vi "VI_Info_da_Quadra_Dasboard.vi"() -> (10 "Match_Time":dbl, 12 "Robot_Position":bool, 14 "Scale_L":bool, 15 "Scale_R":bool, 16 "Switch_R":bool, 17 "Switch_L":bool, 19 "Same_Side":bool)   [LabVIEW 2017]
uses:
  <vilib>/Rock Robotics/Network Tables/NT Read String.vi
  <vilib>/Rock Robotics/Network Tables/NT Read Number.vi
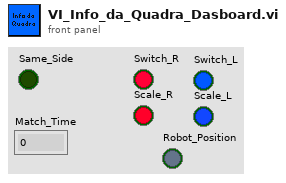
[diagram p1: front panel]
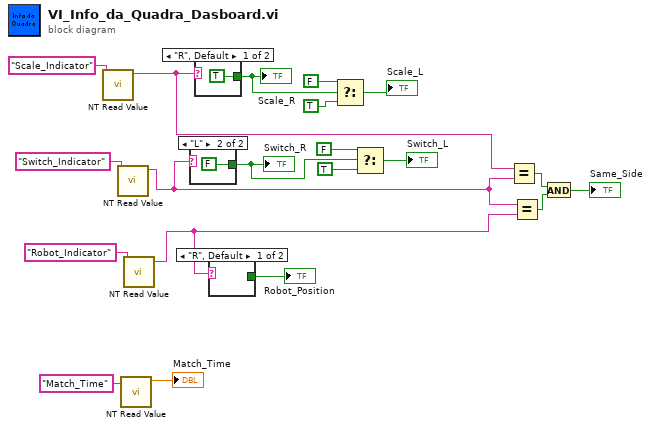
[diagram p0: block diagram]
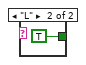
[diagram p2: hidden frame]
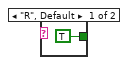
[diagram p3: hidden frame]
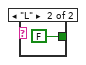
[diagram p4: hidden frame]
diagram:
  n1 = call-poly <vilib>:"NT Read Value.vi"("Name"="Scale_Indicator") -> ("String"=w14:string)  [unwired: 9 in, 1 out]
  n2 = call-poly <vilib>:"NT Read Value.vi"("Name"="Switch_Indicator") -> ("String"=w13:string)  [unwired: 9 in, 1 out]
  n3 = call-poly <vilib>:"NT Read Value.vi"("Name"="Match_Time") -> ("Numeric"=→"Match_Time":dbl)  [unwired: 9 in, 1 out]
  n4 = call-poly <vilib>:"NT Read Value.vi"("Name"="Robot_Indicator") -> ("String"=w12:string)  [unwired: 9 in, 1 out]
  n5 = case shown="\"L\"" w13 {
    tunnel: [TRUE FALSE] -> w8
    frame "R", Default {
    }
    frame "L" {
    }
  }
  "Switch_R" <- w8
  n6 = case shown="\"R\", Default" w14 {
    tunnel: [TRUE FALSE] -> w11
    frame "R", Default {
    }
    frame "L" {
    }
  }
  "Scale_R" <- w11
  n7 = case shown="\"R\", Default" w12 {
    tunnel: [_ TRUE] -> w3
    frame "R", Default {
    }
    frame "L" {
    }
  }
  "Robot_Position" <- w3
  n8 = Select(t=FALSE, s=w11, f=TRUE) -> (s? t:f=→"Scale_L":bool)
  n9 = Select(t=FALSE, s=w8, f=TRUE) -> (s? t:f=→"Switch_L":bool)
  n10 = Equal?(x=w14, y=w13) -> (x = y?=w16:bool)
  n11 = Equal?(x=w13, y=w12) -> (x = y?=w17:bool)
  n12 = And(x=w16, y=w17) -> (x .and. y?=→"Same_Side":bool)
